vi "Parse Data To Send.vi"(8 "Chosen Image Path":path, 9 "Chosen Text":string, 10 "Chosen Transmission Method":u16(ring)=3 items=["Speaker", "Wire", "Motor", "Touch", "Light", "Solenoid"], 11 "Chosen Data Type":u16(ring) items=["Text File", "Image File", "Image", "Text"]) -> ()   [LabVIEW 2025]
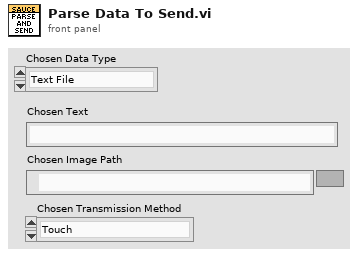
[diagram p1: front panel]
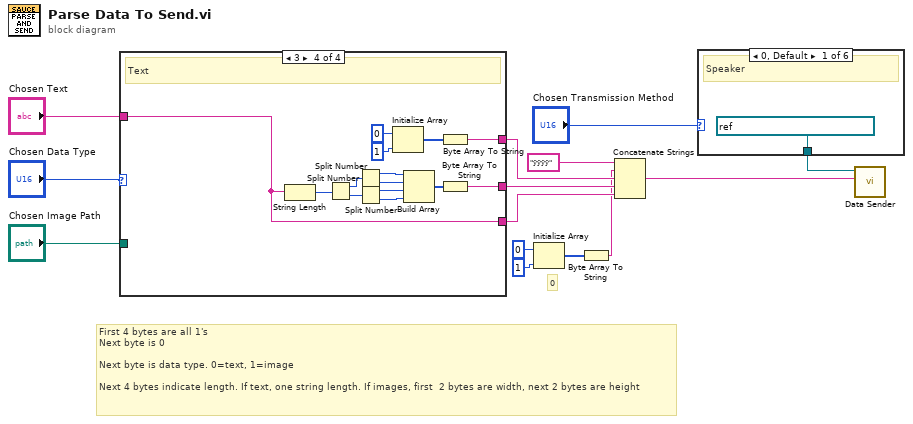
[diagram p0: block diagram]
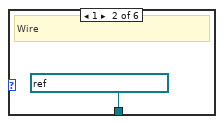
[diagram p2: hidden frame]
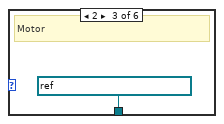
[diagram p3: hidden frame]
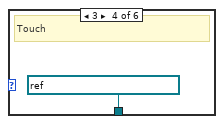
[diagram p4: hidden frame]
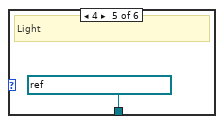
[diagram p5: hidden frame]
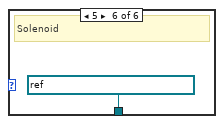
[diagram p6: hidden frame]
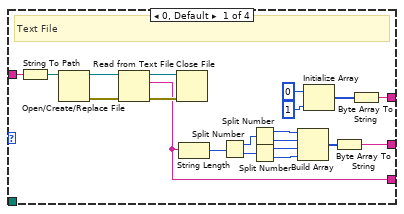
[diagram p7: hidden frame]
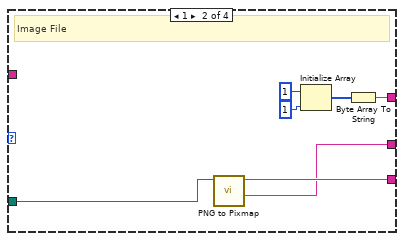
[diagram p8: hidden frame]
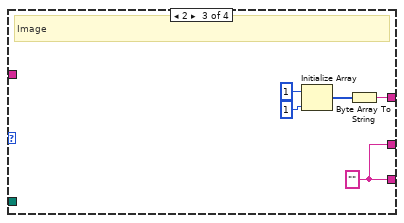
[diagram p9: hidden frame]
diagram:
  # "0"
  # "First 4 bytes are all 1's\nNext byte is 0\n\nNext byte is data type. 0=text, 1=image\n\nNext 4 bytes indicate length. If text, one string length. If images, first  2 bytes are width, next 2 bytes are height"
  n1 = case shown="3" "Chosen Data Type" {
    tunnel: "Chosen Text" -> [w34 _ _ w47]
    tunnel: [w28 w40 w46 w47] -> w9
    tunnel: "Chosen Image Path" -> [_ w41 _ _]
    tunnel: [w23 w35 w42 w58] -> w7
    tunnel: [w27 w39 w46 w48] -> w6
    frame 0, Default {
      # "Text File"
      n2 = String To Path(string=w34) -> (path=w33:path)
      n3 = Open/Create/Replace File(file path (use dialog)=w33) -> (refnum out=w31:refnum<file>, error out=w32:errorcluster)  [unwired: 5 in, 1 out]
      n4 = Read from Text File(file (use dialog)=w31, error in=w32) -> (refnum out=w29:refnum<file>, text=w28:string, error out=w30:errorcluster)  [unwired: 2 in, 1 out]
      n5 = Close File(refnum=w29, error in=w30) -> ()  [unwired: 2 out]
      n6 = String Length(string=w28) -> (length=w15:i32)
      n7 = Split Number(x=w15) -> (hi(x)=w17:u16, lo(x)=w18:u16)
      n8 = Split Number(x=w17) -> (hi(x)=w22:u8, lo(x)=w21:u8)
      n9 = Split Number(x=w18) -> (hi(x)=w19:u8, lo(x)=w20:u8)
      n10 = Build Array(w22, w21, w19, w20) -> (w16:u8[])
      n11 = Initialize Array(0 ("element"), 1 ("dimension size")) -> (w25:i32[])
      n12 = Byte Array To String(unsigned byte array=w16) -> (string=w27:string)
      n13 = Byte Array To String(unsigned byte array=w25) -> (string=w23:string)
    }
    frame 1 {
      # "Image File"
      n14 = call "PNG to Pixmap.vi"("path to PNG file"=w41) -> ("Size"=w39:string, "String"=w40:string)  [unwired: 9 in]
      n15 = Initialize Array(1 ("element"), 1 ("dimension size")) -> (w37:i32[])
      n16 = Byte Array To String(unsigned byte array=w37) -> (string=w35:string)
    }
    frame 2 {
      w46 = "" ("Chosen Text")
      # "Image"
      n17 = Initialize Array(1 ("element"), 1 ("dimension size")) -> (w44:i32[])
      n18 = Byte Array To String(unsigned byte array=w44) -> (string=w42:string)
    }
    frame 3 {
      # "Text"
      n19 = String Length(string=w47) -> (length=w56:i32)
      n20 = Split Number(x=w56) -> (hi(x)=w54:u16, lo(x)=w53:u16)
      n21 = Split Number(x=w54) -> (hi(x)=w49:u8, lo(x)=w50:u8)
      n22 = Split Number(x=w53) -> (hi(x)=w52:u8, lo(x)=w51:u8)
      n23 = Initialize Array(0 ("element"), 1 ("dimension size")) -> (w59:i32[])
      n24 = Build Array(w49, w50, w52, w51) -> (w55:u8[])
      n25 = Byte Array To String(unsigned byte array=w59) -> (string=w58:string)
      n26 = Byte Array To String(unsigned byte array=w55) -> (string=w48:string)
    }
  }
  n27 = Initialize Array(0 ("element"), 1 ("dimension size")) -> (w3:i32[])
  n28 = Byte Array To String(unsigned byte array=w3) -> (string=w1:string)
  n29 = Concatenate Strings("ÿÿÿÿ" ("string"), w1, w7, w6, w9) -> (w8:string)
  n30 = case shown="0, Default" "Chosen Transmission Method" {
    tunnel: [refnum<visa-resource-name> "SPEAKER_TRANSMITTER" ("VISA resource name") refnum<visa-resource-name> "WIRE_TRANSMITTER" ("VISA resource name") refnum<visa-resource-name> "MOTOR_TRANSMITTER" ("VISA resource name") refnum<visa-resource-name> "TOUCH_TRANSMITTER" ("VISA resource name") refnum<visa-resource-name> "LIGHT_TRANSMITTER" ("VISA resource name") refnum<visa-resource-name> "SOLENOID_TRANSMITTER" ("VISA resource name")] -> w10
    frame 0, Default {
      # "Speaker"
    }
    frame 1 {
      # "Wire"
    }
    frame 2 {
      # "Motor"
    }
    frame 3 {
      # "Touch"
    }
    frame 4 {
      # "Light"
    }
    frame 5 {
      # "Solenoid"
    }
  }
  n31 = call "Data Sender.vi"("String To Send"=w8, "VISA resource name"=w10) -> ()  [unwired: 9 in, 1 out]
